vi "ChromaBuildCodeStr.vi"(10 "Hex_input":u64=9984, 11 "Enum_datatype":enum16{"1byte", "2byte", "4byte"}(ring)) -> (2 "Array":u8[](array[numeric]) format="%x", 3 "data string":string)   [LabVIEW 2016]
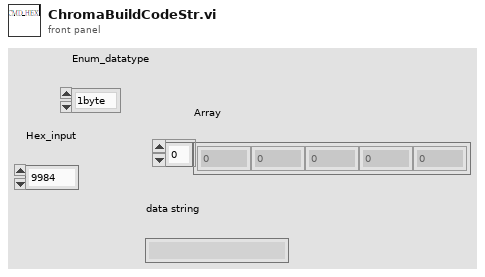
[diagram p1: front panel]
types:
  T1 = enum16{"big-endian, network order", "native, host order", "little-endian"}
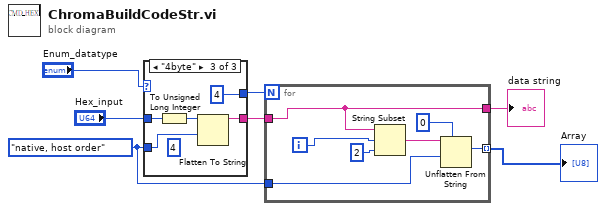
[diagram p0: block diagram]
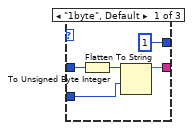
[diagram p2: hidden frame]
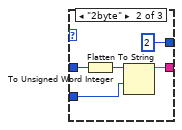
[diagram p3: hidden frame]
diagram:
  w1 = T1."native, host order" ("byte order (0:big-endian, network order)")
  n1 = case shown="\"4byte\"" "Enum_datatype" {
    tunnel: "Hex_input" -> [w12 w17 w22]
    tunnel: w1 -> [w11 w15 w19]
    tunnel: [w9 w14 w20] -> w5
    tunnel: [1 2 4] -> w4
    frame "1byte", Default {
      n2 = To Unsigned Byte Integer(number=w12) -> (unsigned 8bit integer=w10:u8)
      n3 = Flatten To String(anything=w10, byte order (0:big-endian, network order)=w11) -> (data string=w9:string)  [unwired: 2 in, 2 out]
    }
    frame "2byte" {
      n4 = To Unsigned Word Integer(number=w17) -> (unsigned 16bit integer=w16:u16)
      n5 = Flatten To String(anything=w16, byte order (0:big-endian, network order)=w15) -> (data string=w14:string)  [unwired: 2 in, 2 out]
    }
    frame "4byte" {
      (unwired) 4
      n6 = To Unsigned Long Integer(number=w22) -> (unsigned 32bit integer=w21:u32)
      n7 = Flatten To String(anything=w21, byte order (0:big-endian, network order)=w19) -> (data string=w20:string)  [unwired: 2 in, 2 out]
    }
  }
  n8 = for {
    N: w4 -> [_]
    tunnel: w5 -> [w28]
    tunnel: [w28] -> w3
    tunnel: [w25] -> w2 mode=indexing
    tunnel: w1 -> [w24]
    i -> [w23]
    n9 = String Subset(string=w28, offset (0)=w23, length (rest)=2) -> (substring=w27:string)
    n10 = Unflatten From String(type=u8 0, binary string=w27, byte order (0:big-endian, network order)=w24) -> (value=w25:u8)  [unwired: 2 in, 2 out]
  }
  "data string" <- w3
  "Array" <- w2
